vi "Write Command and Read.vi"(5 "Wait before read (0ms)":u32, 6 "error in (no error)":errorcluster, 7 "Bytes to read (100)":u32=100, 8 "Command":string, 9 "VISA resource name":refnum<visa-resource-name>="COM5") -> (0 "error out":errorcluster, 2 "Returned string":string, 3 "VISA resource name out":refnum<visa-resource-name>="COM5")   [LabVIEW 2019, in "Newport ESP301.lvlib"]
uses:
  Newport ESP301.lvlib
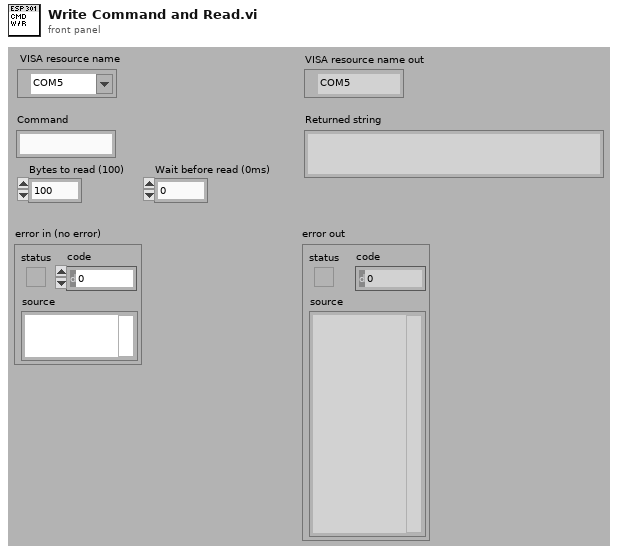
[diagram p1: front panel]
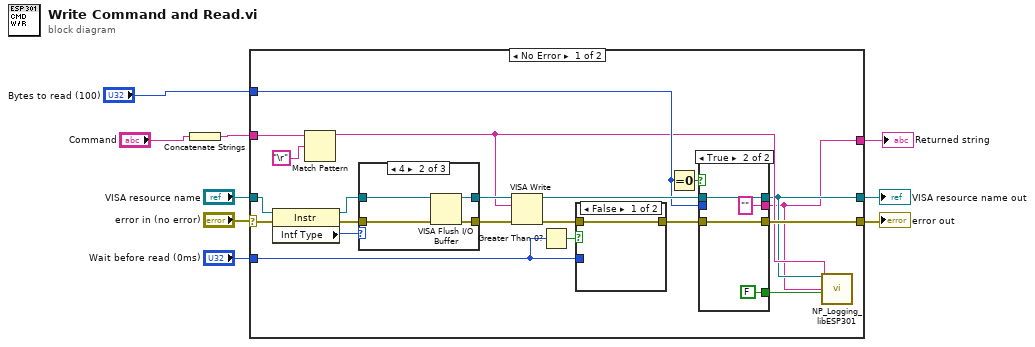
[diagram p0: block diagram]
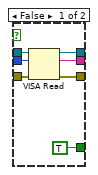
[diagram p4: hidden frame]
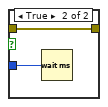
[diagram p5: hidden frame]
diagram:
  n1 = Concatenate Strings("Command") -> (w1:string)
  n2 = case shown="No Error" "error in (no error)" {
    selector: "error in (no error)" -> [w18 w54]
    tunnel: [w30 w54] -> w8
    tunnel: "VISA resource name" -> [w19 w53]
    tunnel: [w13 w53] -> w6
    tunnel: w1 -> [w17 _]
    tunnel: "Bytes to read (100)" -> [w22 _]
    tunnel: [w12 _] -> w4
    tunnel: "Wait before read (0ms)" -> [w24 _]
    frame No Error {
      n3 = property class="Instr"(reference=w19, error in=w18) -> (reference out=w11:refnum<visa-resource-name>, error out=w10:errorcluster, "Intf Type"=w20:u16)
      n4 = Match Pattern(string=w17, regular expression="\r") -> (before substring=w14:string)  [unwired: 4 out]
      n5 = case shown="4" w20 {
        tunnel: w11 -> [w32 w34 w38]
        tunnel: [w32 w33 w38] -> w28
        tunnel: w10 -> [w31 w36 w37]
        tunnel: [w31 w35 w37] -> w27
        frame 1 {
        }
        frame 4 {
          n6 = VISA Flush I/O Buffer(VISA resource name=w34, error in (no error)=w36) -> (VISA resource name out=w33:refnum<visa-resource-name>, error out=w35:errorcluster)  [unwired: 1 out]
        }
        frame Default {
        }
      }
      n7 = VISA Write(VISA resource name=w28, write buffer=w14, error in (no error)=w27) -> (VISA resource name out=w29:refnum<visa-resource-name>, error out=w26:errorcluster)  [unwired: 1 out]
      n8 = Greater Than 0?(x=w24) -> (x > 0?=w23:bool)
      n9 = case shown="False" w23 {
        tunnel: w26 -> [w50 w52]
        tunnel: [w50 w52] -> w25
        tunnel: w24 -> [_ w51]
        frame False {
        }
        frame True {
          n10 = Wait (ms)(milliseconds to wait=w51) -> ()  [unwired: 1 out]
        }
      }
      n11 = Equal To 0?(x=w22) -> (x = 0?=w21:bool)
      n12 = case shown="True" w21 {
        tunnel: [w45 w49] -> w30
        tunnel: w29 -> [w44 w48]
        tunnel: [w43 w48] -> w13
        tunnel: w22 -> [w42 _]
        tunnel: [w41 "" ("read buffer")] -> w12
        tunnel: w25 -> [w40 w49]
        tunnel: [TRUE ("String 2 Enable (T)") FALSE ("String 2 Enable (T)")] -> w15
        frame False {
          n13 = VISA Read(VISA resource name=w44, byte count=w42, error in (no error)=w40) -> (VISA resource name out=w43:refnum<visa-resource-name>, read buffer=w41:string, error out=w45:errorcluster)  [unwired: 1 out]
        }
        frame True {
        }
      }
      n14 = call "NP_Logging_libESP301.vi"("Instrument Channel"=w13, "String 1 {Write} (in)"=w14, "String 2 {Read} (in)"=w12, "String 2 Enable (T)"=w15) -> ()  [unwired: 8 in, 4 out]
    }
    frame Error {
    }
  }
  "error out" <- w8
  "VISA resource name out" <- w6
  "Returned string" <- w4
